vi "Close.vi"(8 "error in (no error)":errorcluster, 11 "InterfaceLog in":refnum<class "InterfaceLog.lvclass">) -> (0 "error out":errorcluster, 3 "InterfaceLog out":refnum<class "InterfaceLog.lvclass">)   [LabVIEW 2016, in "InterfaceLog.lvclass"]
uses:
  InterfaceLog.lvclass
  InterfaceLog.lvclass/InterfaceLog.ctl
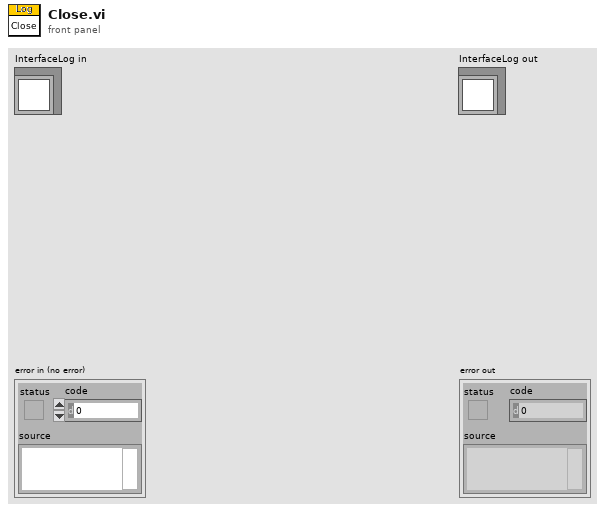
[diagram p1: front panel]
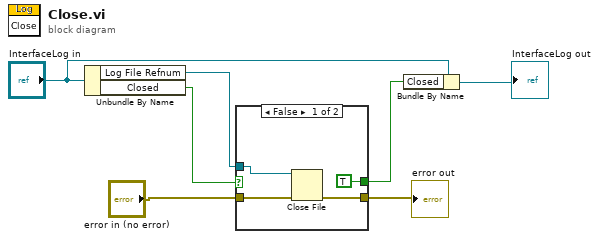
[diagram p0: block diagram]
diagram:
  n1 = Unbundle By Name("InterfaceLog in") -> ("Log File Refnum"=w4:refnum<file>, "Closed"=w5:bool)
  n2 = case shown="False" w5 {
    selector: w5 -> [_ w13]
    tunnel: w4 -> [w11 _]
    tunnel: "error in (no error)" -> [w10 w12]
    tunnel: [w9 w12] -> w2
    tunnel: [TRUE w13] -> w1
    frame False {
      n3 = Close File(refnum=w11, error in=w10) -> (error out=w9:errorcluster)  [unwired: 1 out]
    }
    frame True {
    }
  }
  "error out" <- w2
  n4 = Bundle By Name(cluster="InterfaceLog in", "Closed"=w1) -> (→"InterfaceLog out":refnum<class "InterfaceLog.lvclass">)
